vi "Configure CheckSum.vi"(0 "VISA resource name":refnum<visa-resource-name>, 5 "Enable CheskSum? (Off)":bool, 11 "error in (no error)":errorcluster) -> (4 "VISA resource name out":refnum<visa-resource-name>, 15 "error out":errorcluster)   [LabVIEW 2020, in "Yokogawa GX Series.lvlib"]
doc: "This VI sets the alarm hysteresis for <B>DX1000/DX2000 series</B>.\nThis VI can be used on Basic Setting Mode at the <B>Set Execution Mode.VI</B>.\n\nAlarm settings on computation channels can be specified on models with the /M1 or /PM1 math option.\nAlarm settings on external input channels can be specified on models with the /MC1 external input channel option."
uses:
  <instrlib>/Yokogawa GX Series/Yokogawa GX Series.lvlib
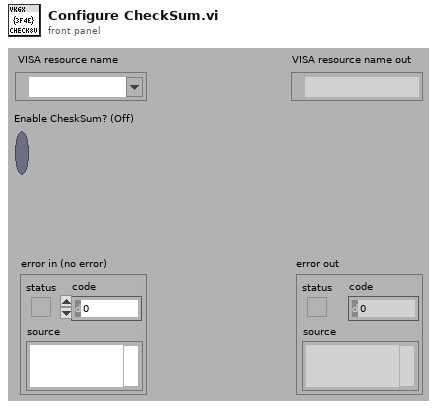
[diagram p1: front panel]
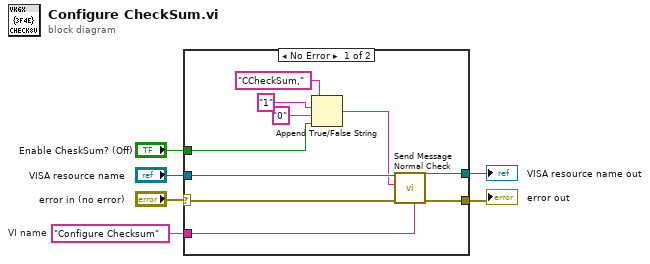
[diagram p0: block diagram]
diagram:
  w6 = "Configure Checksum"  # VI name
  n1 = case shown="No Error" "error in (no error)" {
    selector: "error in (no error)" -> [w7 w17]
    tunnel: w6 -> [w16 _]
    tunnel: [w15 w18] -> w5
    tunnel: [w14 w17] -> w4
    tunnel: "VISA resource name" -> [w13 w18]
    tunnel: "Enable CheskSum? (Off)" -> [w10 _]
    frame No Error {
      n2 = Append True/False String(1:w10, 2:"0", 3:"1", 4:"CCheckSum,") -> (0:w11:string)
      n3 = call <instrlib>:"Send Message Normal Check.vi"("Source (\"\")"=w16, "error in (no error)"=w7, "Send Message (\"\")"=w11, "VISA resource name"=w13) -> ("error out"=w14:errorcluster, "VISA resource name out"=w15:refnum<visa-resource-name>)  [unwired: 2 in, 4 out]
    }
    frame Error {
    }
  }
  "error out" <- w4
  "VISA resource name out" <- w5
